vi "Library VI Children Data.vi"(7 "Destination":path, 8 "Error In":errorcluster, 11 "Library In":refnum<vi>) -> (0 "Error Out":errorcluster, 2 "Data":refnum<class "Map.lvclass">[](array[class]), 3 "Library Out":refnum<vi>)   [LabVIEW 2018, in "Scripts.lvlib"]
uses:
  Scripts.lvlib
  Toolkit/Data/Map/Map.lvclass
  Toolkit/Data/Map/Support/From String.vi
  Toolkit/Data/Map/Support/From Map Array.vi
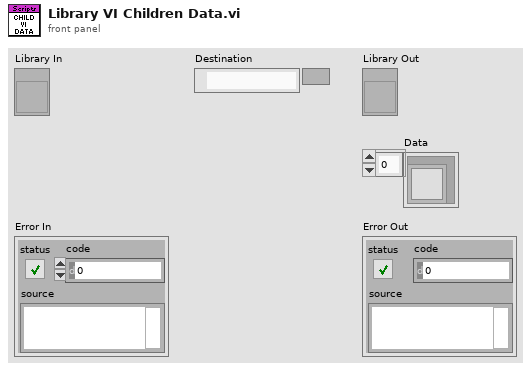
[diagram p1: front panel]
types:
  T1 = enum32{"invalid scope", "public", "private", "protected", "community"}
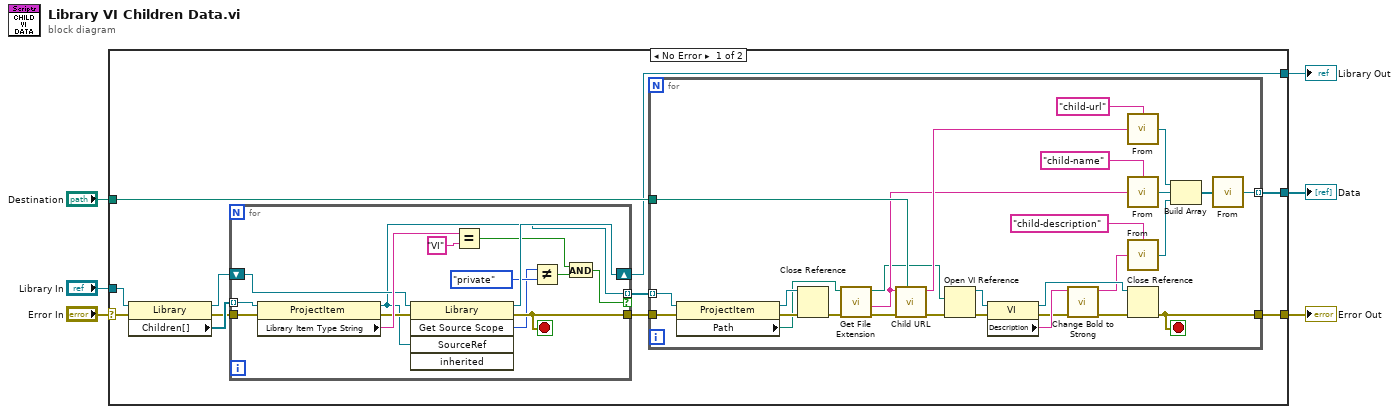
[diagram p0: block diagram]
diagram:
  n1 = case shown="No Error" "Error In" {
    selector: "Error In" -> [w13 w61]
    tunnel: [w17 w61] -> w6
    tunnel: "Destination" -> [w15 _]
    tunnel: "Library In" -> [w14 w60]
    tunnel: [w7 w60] -> w3
    tunnel: [w16 _] -> w2
    frame No Error {
      n2 = property class="Library"(reference=w14, error in=w13) -> (reference out=w8:refnum<vi>, error out=w11:errorcluster, "Children[]"=w12:refnum<vi>[])
      n3 = for {
        tunnel: w12 -> [w31] mode=indexing
        tunnel: w11 -> [w30]
        tunnel: [w22] -> w9 mode=indexing if=w18
        tunnel: [w24] -> w10
        shift-right: [w26] -> w7
        shift-left: w8 -> [w27]
        stop <- w24 stop-if-true
        n4 = property class="ProjectItem"(reference=w31, error in=w30) -> (reference out=w22:refnum<vi>, error out=w25:errorcluster, "Library Item Type String"=w29:string)
        n5 = invoke class="Library" method="Get Source Scope"(reference=w27, error in=w25, "SourceRef"=w22) -> (reference out=w26:refnum<vi>, error out=w24:errorcluster, "GetSourceScope"=w20:T1)  [unwired: 2 in, 2 out]
        n6 = Equal?(x=w29, y="VI") -> (x = y?=w23:bool)
        n7 = Not Equal?(x=w20, y=T1."private" ("Source Scope:Get")) -> (x != y?=w19:bool)
        n8 = And(x=w23, y=w19) -> (x .and. y?=w18:bool)
      }
      n9 = for {
        tunnel: w10 -> [w53]
        tunnel: [w54] -> w16 mode=indexing
        tunnel: [w45] -> w17
        tunnel: w15 -> [w41]
        tunnel: w9 -> [w35] mode=indexing
        stop <- w45 stop-if-true
        n10 = property class="ProjectItem"(reference=w35, error in=w53) -> (reference out=w49:refnum<vi>, error out=w50:errorcluster, "Path"=w48:path)
        n11 = Close Reference(reference=w49, error in (no error)=w50) -> (error out=w47:errorcluster)
        n12 = call <vilib>:"Get File Extension.vi"("error in (no error)"=w47, "file"=w48) -> ("error out"=w44:errorcluster, "filename without extension"=w40:string, "dup file"=w33:path)  [unwired: 5 in, 2 out]
        n13 = call "Child URL.vi"("Destination"=w41, "Error In"=w44, "Name"=w40) -> ("Error Out"=w43:errorcluster, "Child URL"=w42:string)  [unwired: 7 in]
        n14 = Open VI Reference(vi path=w33, error in (no error)=w43) -> (vi reference=w32:refnum<vi>, error out=w34:errorcluster)  [unwired: 4 in]
        n15 = property class="VI"(reference=w32, error in=w34) -> (reference out=w46:refnum<vi>, error out=w38:errorcluster, "Description"=w39:string)
        n16 = call "Change Bold to Strong.vi"("Error In"=w38, "Bold Description"=w39) -> ("Error Out"=w37:errorcluster, "Strong Description"=w36:string)  [unwired: 8 in]
        n17 = call-poly "From.vi"("Value"=w42, "Key"="child-url") -> ("Map"=w57:refnum<class "Map.lvclass">)
        n18 = call-poly "From.vi"("Value"=w40, "Key"="child-name") -> ("Map"=w56:refnum<class "Map.lvclass">)
        n19 = call-poly "From.vi"("Value"=w36, "Key"="child-description") -> ("Map"=w51:refnum<class "Map.lvclass">)
        n20 = Close Reference(reference=w46, error in (no error)=w37) -> (error out=w45:errorcluster)
        n21 = Build Array(w57, w56, w51) -> (w55:refnum<class "Map.lvclass">[])
        n22 = call-poly "From.vi"("Maps"=w55) -> ("Map"=w54:refnum<class "Map.lvclass">)  [unwired: 1 in]
      }
    }
    frame Error {
    }
  }
  "Error Out" <- w6
  "Library Out" <- w3
  "Data" <- w2
